vi "Test CAN Logger with TDMS.vi"() -> ()   [LabVIEW 2014]
uses:
  <vilib>/RioEmbeddedCAN/RioEmbeddedCAN.llb/CANFrameControl.ctl
  <vilib>/NI_Real-Time Target Support.lvlib
  <vilib>/Utility/RT CPU Load.ctl
panel:
  out "Logged Messages/second":dbl
  out "Array":T3(array[cluster]) {"CAN frame"."type" items=["CAN Data", "CAN Remote"]; "CAN frame"."identifier" format="%.0x"; "CPU loads"."ISR (%)" format="%#.2f"; "CPU loads"."Idle (%)" format="%#.2f"; "CPU loads"."Background (%)" format="%#.2f"; "CPU loads"."Normal (%)" format="%#.2f"; "CPU loads"."Above Normal (%)" format="%#.2f"; "CPU loads"."High (%)" format="%#.2f"; "CPU loads"."Timed Structures (%)" format="%#.2f"; "CPU loads"."Time Critical (%)" format="%#.2f"; "CPU loads"."Total (%)" format="%#.2f"}
  in  "Boolean":bool
  out "error out":errorcluster
  out "index":i32
  in  "baud rate (125000 bps)":u32=1000000
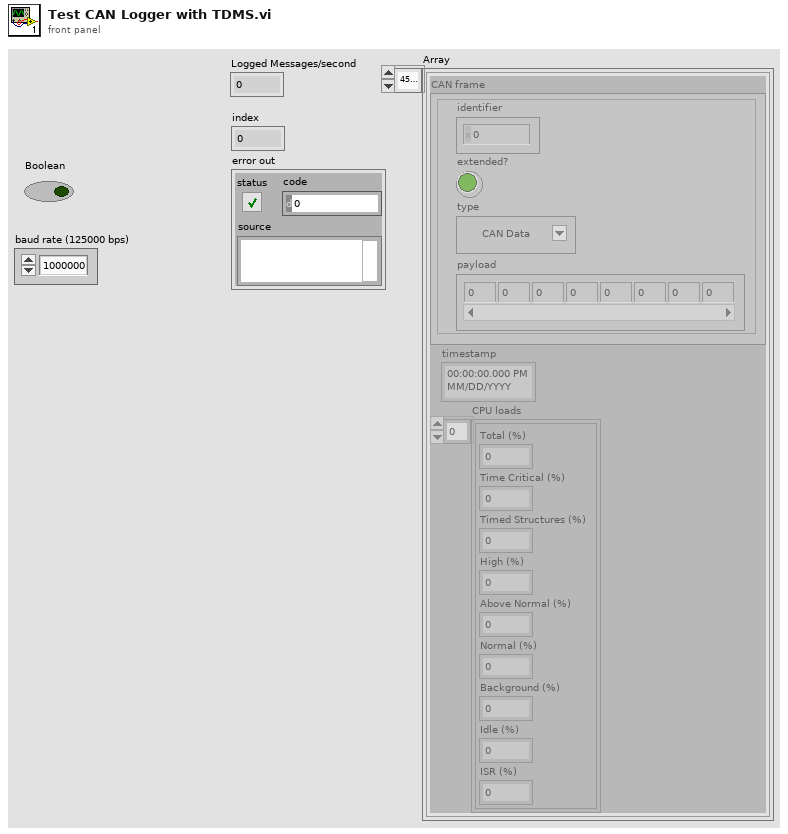
[diagram p1: front panel]
types:
  T1 = typedef "CANFrameControl.ctl" = cluster{"identifier":u32, "extended?":bool, "type":u8, "payload":u8[]}
  T2 = typedef "NI_Real-Time Target Support.lvlib/RT CPU Load.ctl" = cluster{"Total (%)":dbl, "Time Critical (%)":dbl, "Timed Structures (%)":dbl, "High (%)":dbl, "Above Normal (%)":dbl, "Normal (%)":dbl, "Background (%)":dbl, "Idle (%)":dbl, "ISR (%)":dbl}
  T3 = cluster{"CAN frame":T1, "timestamp":timestamp, "CPU loads":T2[]}[]
  T4 = enum16{"open", "open or create", "create or replace", "create", "open (read-only)"}
  T5 = cluster{"CAN frame":T1, "timestamp":timestamp, "CPU loads":T2[]}
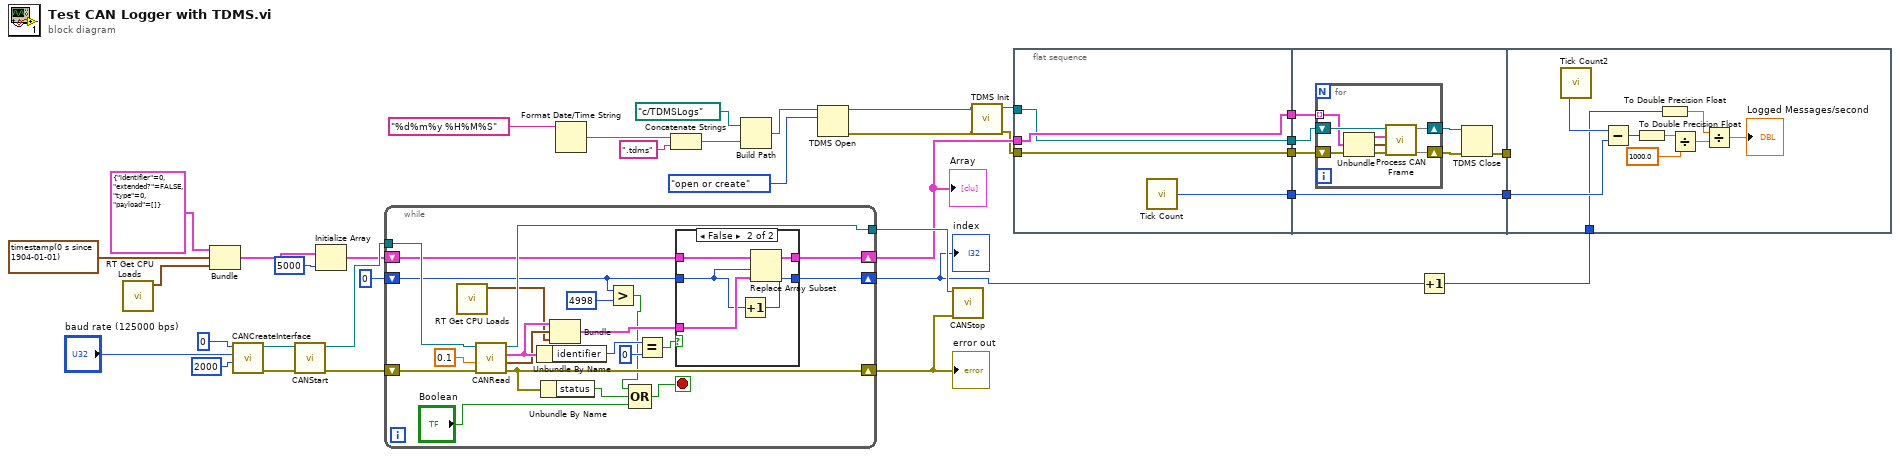
[diagram p0: block diagram]
diagram:
  n1 = call <vilib>:"RT Get CPU Loads.vi"() -> ("CPU loads"=w10:T2[])  [unwired: 10 in, 1 out]
  n2 = Bundle("CAN frame"=T1 {"identifier"=0, "extended?"=FALSE, "type"=0, "payload"=[]}, "timestamp"=timestamp(0 s since 1904-01-01), "CPU loads"=w10) -> (w15:T5)  [unwired: 1 in]
  n3 = call <vilib>:"CANCreateInterface.vi"("receive queue size (5)"=u32 2000, "baud rate (125000 bps)"="baud rate (125000 bps)", "interface index"=u32 0) -> ("error out"=w36:errorcluster, "interface object out"=w35:refnum<k20>)  [unwired: 7 in]
  n4 = call <vilib>:"CANStart.vi"("error in (no error)"=w36, "interface object in"=w35) -> ("error out"=w26:errorcluster, "interface object out"=w34:refnum<k20>)  [unwired: 8 in]
  n5 = Initialize Array(w15, 5000 ("dimension size")) -> (w29:T3)
  n6 = while {
    tunnel: w34 -> [w57]
    tunnel: [w56] -> w33
    shift-right: [w51] -> w14
    shift-left: w29 -> [w55]
    shift-right: [w52] -> w7
    shift-left: 0 ("index") -> [w42]
    shift-right: [w48] -> w32
    shift-left: w26 -> [w49]
    stop <- w37 stop-if-true
    n7 = call <vilib>:"RT Get CPU Loads.vi"() -> ("CPU loads"=w44:T2[])  [unwired: 10 in, 1 out]
    n8 = call <vilib>:"CANRead.vi"("error in (no error)"=w49, "timeout (0 s)"=0.1, "interface object in"=w57) -> ("error out"=w48:errorcluster, "timestamp"=w46:timestamp, "CAN frame"=w47:T1, "interface object out"=w56:refnum<k20>)  [unwired: 5 in]
    n9 = Unbundle By Name(w47) -> ("identifier"=w54:u32)
    n10 = Unbundle By Name(w48) -> ("status"=w39:bool)
    n11 = Bundle("CAN frame"=w47, "timestamp"=w46, "CPU loads"=w44) -> (w45:T5)  [unwired: 1 in]
    n12 = Greater?(x=w42, y=4998) -> (0:w40:bool)
    n13 = Compound Arithmetic op=OR(w40, w39, "Boolean") -> (w37:bool)
    n14 = Equal?(x=w54, y=u32 0) -> (x = y?=w53:bool)
    n15 = case shown="False" w53 {
      tunnel: w55 -> [w59 w62]
      tunnel: [w59 w63] -> w51
      tunnel: w42 -> [w58 w60]
      tunnel: w45 -> [_ w61]
      tunnel: [w58 w64] -> w52
      frame True {
      }
      frame False {
        n16 = Increment(x=w60) -> (x+1=w64:i32)
        n17 = Replace Array Subset(array=w62, new element=w61, index=w60) -> (w63:T3)
      }
    }
  }
  "index" <- w7
  "error out" <- w32
  "Array" <- w14
  n18 = Format Date/Time String(time format string (%c)="%d%m%y %H%M%S") -> (date/time string=w21:string)  [unwired: 2 in]
  n19 = Concatenate Strings(w21, ".tdms" ("string")) -> (w23:string)
  n20 = Build Path(base path=path "c:/TDMSLogs", name or relative path=w23) -> (appended path=w22:path)
  n21 = TDMS Open(10:T4."open or create" ("operation (0:open)"), 11:w22) -> (0:w4:errorcluster, 3:w5:refnum<k34>)  [unwired: 5 in]
  n22 = call <vilib>:"CANStop.vi"("error in (no error)"=w32, "interface object in"=w33) -> ()  [unwired: 8 in, 2 out]
  n23 = call "TDMS Init.vi"("error in (no error)"=w4, "tdms file"=w5) -> ("error out"=w2:errorcluster, "tdms file out"=w3:refnum<k34>)  [unwired: 8 in]
  n24 = flat-sequence {
    tunnel: w2 -> [w66]
    tunnel: w3 -> [w67]
    tunnel: w14 -> [w68]
    tunnel: [w68] -> w13
    tunnel: [w67] -> w12
    tunnel: [w66] -> w11
    tunnel: [w65] -> w8
    tunnel: w13 -> [w75]
    tunnel: w12 -> [w74]
    tunnel: w11 -> [w73]
    tunnel: [w72] -> w9
    tunnel: w8 -> [w72]
    tunnel: [w69] -> w1
    tunnel: w9 -> [w91]
    tunnel: w6 -> [w84]
    tunnel: w1 -> [_]
    frame #0 {
      n25 = call "Tick Count"() -> ("Tick Count(mSec)"=w65:u32)
    }
    frame #1 {
      n26 = for {
        tunnel: w75 -> [w80] mode=indexing
        shift-right: [w77] -> w70
        shift-left: w74 -> [w82]
        shift-right: [w76] -> w71
        shift-left: w73 -> [w81]
        n27 = Unbundle(w80) -> ("CAN frame"=w78:T1, "timestamp"=w79:timestamp)  [unwired: 1 out]
        n28 = call "Process CAN Frame.vi"(8:w81, 9:w79, "CAN frame"=w78, 11:w82) -> (0:w76, 3:w77)  [unwired: 6 in]
      }
      n29 = TDMS Close(8:w71, 11:w70) -> (0:w69:errorcluster)  [unwired: 1 out]
    }
    frame #2 {
      n30 = call "Tick Count2"() -> ("Tick Count(mSec)"=w90:u32)
      n31 = Subtract(x=w90, y=w91) -> (x-y=w89:u32)
      n32 = To Double Precision Float(number=w89) -> (double precision float=w88:dbl)
      n33 = To Double Precision Float(number=w84) -> (double precision float=w85:dbl)
      n34 = Divide(x=w88, y=1000.0) -> (x/y=w86:dbl)
      n35 = Divide(x=w85, y=w86) -> (x/y=→"Logged Messages/second":dbl)
    }
  }
  n36 = Increment(x=w7) -> (x+1=w6:i32)
